vi "ConnectAtlas.vi"(8 "error in (no error)":errorcluster) -> (1 "Atlas connection":bool=TRUE, 2 "AtlatsStat":string[](array[string]), 3 "Laser status":bool[](array[boolean]))   [LabVIEW 2019]
uses:
  <vilib>/regexp/Match Regular Expression.xnode
panel:
  out "body":string
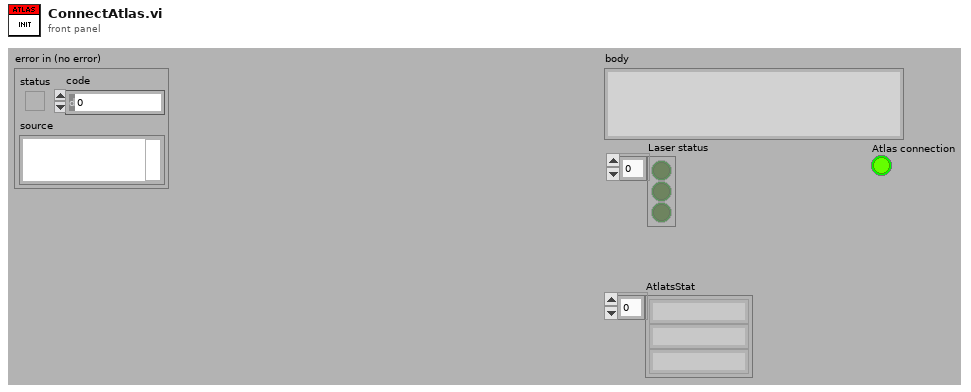
[diagram p1: front panel]
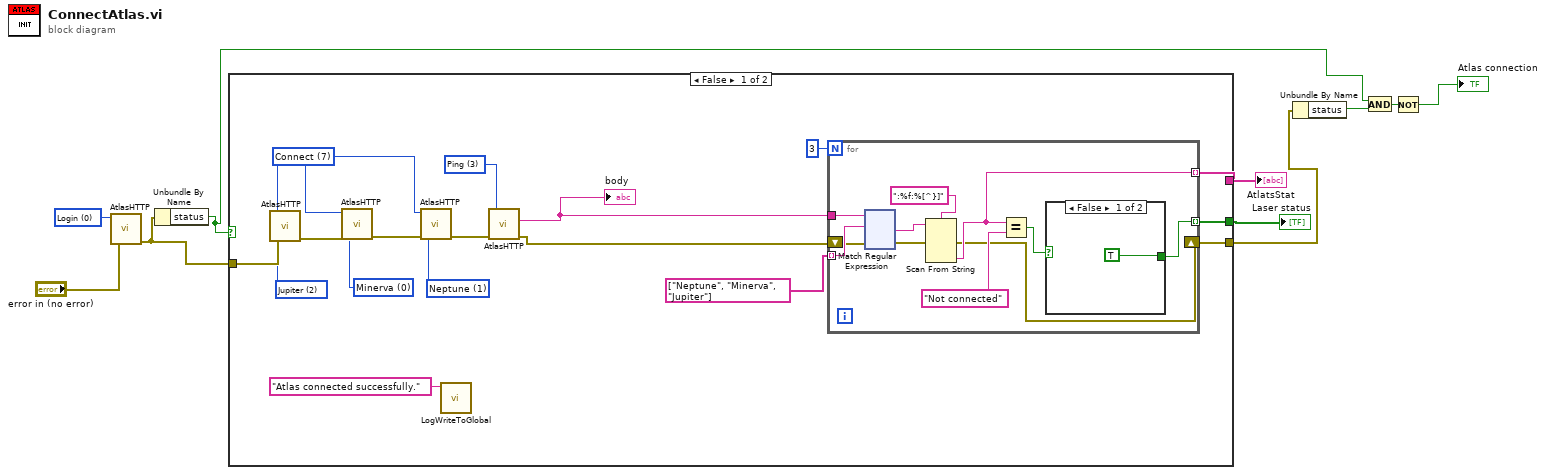
[diagram p0: block diagram]
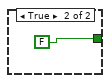
[diagram p2: hidden frame]
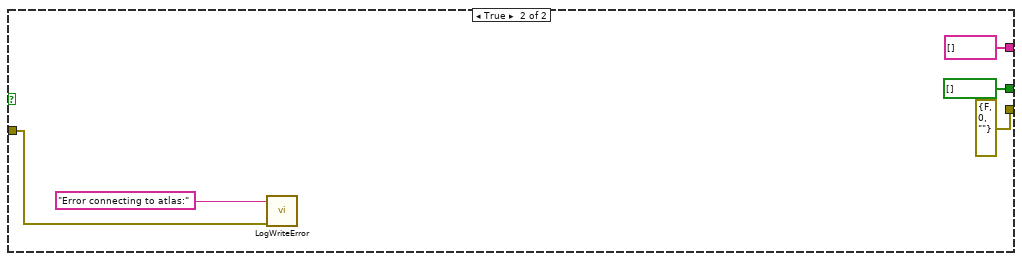
[diagram p3: hidden frame]
diagram:
  w10 = u16 0 items=["Login", "Logout", "get_laser_names", "Ping", "Unlock", "Lock171", "Lock174", "Connect", "Disconnect"] ("Command")
  n1 = call "AtlasHTTP.vi"("error in (no error)"="error in (no error)", "Command"=w10) -> ("error out"=w7:errorcluster)  [unwired: 6 in, 1 out]
  n2 = Unbundle By Name(w7) -> ("status"=w3:bool)
  n3 = case shown="False" w3 {
    tunnel: w7 -> [w27 w153]
    tunnel: [w17 bool[] []] -> w9
    tunnel: [w16 string[] []] -> w8
    tunnel: [w11 errorcluster {"status"=FALSE, "code"=0, "source"=""} ("error out")] -> w5
    frame False {
      w19 = u16 3 items=["Login", "Logout", "get_laser_names", "Ping", "Unlock", "Lock171", "Lock174", "Connect", "Disconnect"] ("Command")
      w21 = u16 1 items=["Minerva", "Neptune", "Jupiter"] ("Laser")
      w22 = u16 0 items=["Minerva", "Neptune", "Jupiter"] ("Laser")
      w26 = u16 2 items=["Minerva", "Neptune", "Jupiter"] ("Laser")
      w23 = u16 7 items=["Login", "Logout", "get_laser_names", "Ping", "Unlock", "Lock171", "Lock174", "Connect", "Disconnect"] ("Command")
      n4 = call "AtlasHTTP.vi"("error in (no error)"=w27, "Laser"=w26, "Command"=w23) -> ("error out"=w25:errorcluster)  [unwired: 5 in, 1 out]
      n5 = call "AtlasHTTP.vi"("error in (no error)"=w25, "Laser"=w22, "Command"=w23) -> ("error out"=w24:errorcluster)  [unwired: 5 in, 1 out]
      n6 = call "AtlasHTTP.vi"("error in (no error)"=w24, "Laser"=w21, "Command"=w23) -> ("error out"=w20:errorcluster)  [unwired: 5 in, 1 out]
      n7 = call "LogWriteToGlobal.vi"("in string"="Atlas connected successfully.") -> ()  [unwired: 11 in]
      n8 = call "AtlasHTTP.vi"("error in (no error)"=w20, "Command"=w19) -> ("error out"=w12:errorcluster, "body"=w18:string)  [unwired: 6 in]
      "body" <- w18
      n9 = for {
        N: 3 -> [_]
        tunnel: w18 -> [w38]
        tunnel: string[] ["Neptune", "Minerva", "Jupiter"] -> [w36] mode=indexing
        tunnel: [w33] -> w17 mode=indexing
        tunnel: [w32] -> w16 mode=indexing
        shift-right: [w28] -> w11
        shift-left: w12 -> [w30]
        n10 = xnode "Match Regular Expression"("input string"=w38, "regular expression"=w36, "error in"=w30) -> ("after match"=w37:string, "error out"=w29:errorcluster)  [unwired: 3 in, 3 out]
        n11 = Scan From String(format string=":%f:%[^}]", input string=w37, error in=w29) -> (error out=w28:errorcluster, output 2=w32:string)  [unwired: 4 in, 2 out]
        n12 = Equal?(x=w32, y="Not connected") -> (x = y?=w35:bool)
        n13 = case shown="False" w35 {
          tunnel: [TRUE FALSE] -> w33
          frame False {
          }
          frame True {
          }
        }
      }
    }
    frame True {
      n14 = call "LogWriteError.vi"("error constant"=w153, "in string"="Error connecting to atlas:") -> ()  [unwired: 10 in]
    }
  }
  "Laser status" <- w9
  "AtlatsStat" <- w8
  n15 = Unbundle By Name(w5) -> ("status"=w4:bool)
  n16 = And(x=w3, y=w4) -> (x .and. y?=w2:bool)
  n17 = Not(x=w2) -> (.not. x?=→"Atlas connection":bool)
